vi "read_continuosData.vi"(8 "error in":errorcluster, 11 "DirPath":path) -> (0 "error out":errorcluster, 2 "CurrenMeters":cluster{"Array":timestamp[], "Array":dbl[]}[](array[cluster]), 3 "StrainGauges":cluster{"Array":timestamp[], "Array":dbl[]}[](array[cluster]))   [LabVIEW 2016]
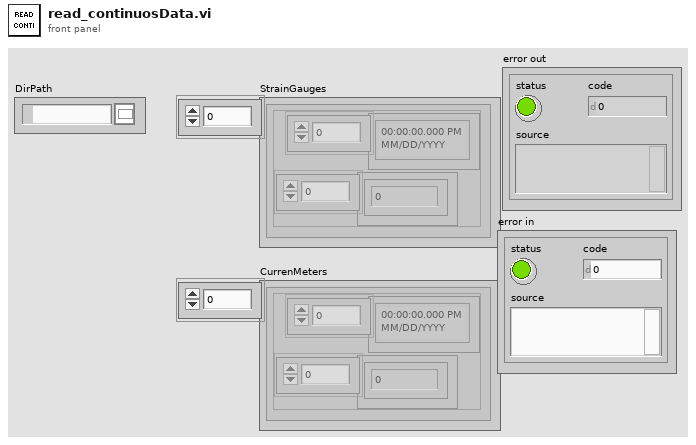
[diagram p1: front panel]
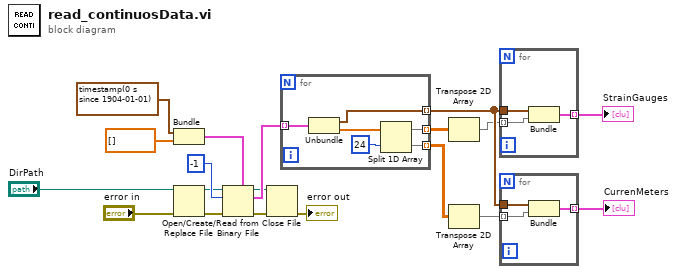
[diagram p0: block diagram]
diagram:
  n1 = Bundle(timestamp(0 s since 1904-01-01), dbl[] []) -> (w11:cluster{timestamp, dbl[]})  [unwired: 1 in]
  n2 = Open/Create/Replace File(file path (use dialog)="DirPath", error in="error in") -> (refnum out=w4:refnum<file>, error out=w5:errorcluster)  [unwired: 4 in, 1 out]
  n3 = Read from Binary File(5:w11, 8:w5, 10:-1 ("count (1)"), 11:w4) -> (0:w8:errorcluster, 2:w12:cluster{timestamp, dbl[]}[], 3:w7:refnum<file>)  [unwired: 2 in, 1 out]
  n4 = Close File(refnum=w7, error in=w8) -> (error out=→"error out":errorcluster)  [unwired: 1 out]
  n5 = for {
    tunnel: w12 -> [w25] mode=indexing
    tunnel: [w22] -> w13 mode=indexing
    tunnel: [w21] -> w15 mode=indexing
    tunnel: [w20] -> w18 mode=indexing
    n6 = Unbundle(w25) -> (w20:timestamp, w24:dbl[])
    n7 = Split 1D Array(array=w24, index=24) -> (first subarray=w22:dbl[], second subarray=w21:dbl[])
  }
  n8 = Transpose 2D Array(2D array=w13) -> (transposed array=w14:dbl[][])
  n9 = Transpose 2D Array(2D array=w15) -> (transposed array=w17:dbl[][])
  n10 = for {
    tunnel: w14 -> [w28] mode=indexing
    tunnel: w18 -> [w27]
    tunnel: [w26] -> w16 mode=indexing
    n11 = Bundle(w27, w28) -> (w26:cluster{timestamp[], dbl[]})  [unwired: 1 in]
  }
  "StrainGauges" <- w16
  n12 = for {
    tunnel: w17 -> [w31] mode=indexing
    tunnel: w18 -> [w30]
    tunnel: [w29] -> w19 mode=indexing
    n13 = Bundle(w30, w31) -> (w29:cluster{timestamp[], dbl[]})  [unwired: 1 in]
  }
  "CurrenMeters" <- w19
